vi "read4Byte Tx.vi"(7 "address":u16, 8 "error in (no error)":errorcluster, 9 "id":u8, 10 "protocol_version":i32, 11 "port_num":i32) -> (0 "error out":errorcluster)   [LabVIEW 2022 SP3, in "dxl.lvlib"]
doc: "WINDECLSPEC void read4ByteTx (int port_num, int protocol_version, uint8_t id, uint16_t address);"
uses:
  dxl.lvlib
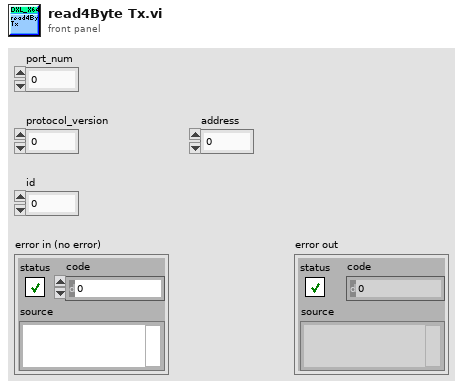
[diagram p1: front panel]
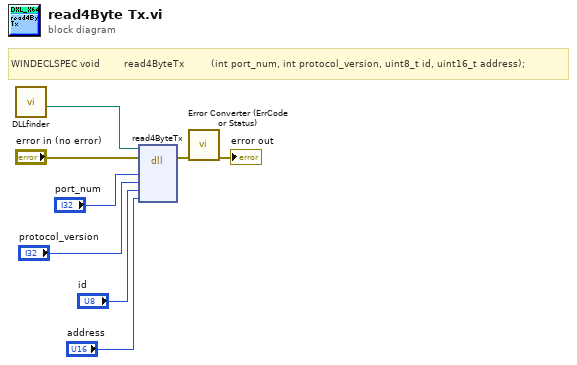
[diagram p0: block diagram]
diagram:
  # "WINDECLSPEC void        read4ByteTx         (int port_num, int protocol_version, uint8_t id, uint16_t address);"
  n1 = call "DLLfinder.vi"() -> ("File Path"=w1:path)  [unwired: 11 in]
  n2 = dll-call lib="C:/EnFlo_Software/ADAM Serial/Instrument drivers/Dynamixel/2nd attempt/Library/dxl_x64_c.*" fn="read4ByteTx"(path in=w1, error in="error in (no error)", "port_num"="port_num", "protocol_version"="protocol_version", "id"="id", "address"="address") -> (error out=w3:errorcluster)  [unwired: 6 in, 1 out]
  n3 = call "Error Converter (ErrCode or Status).vi"("error in (no error)"=w3) -> ("error out"=→"error out":errorcluster)  [unwired: 10 in]
